vi "Format Spreadsheet Header.vi"(10 "Channel Settings":T1[](array[typedef])) -> (2 "Log file header":string)   [LabVIEW 2021, in "Logging.lvlib"]
doc: "Format a starting timestamp and column headings using the channel names from 'Channel Settings'."
uses:
  Logging.lvlib
  Acquisition/Channel Settings.ctl
  Acquisition/IO Device.ctl
  Acquisition/Acquisition.lvlib
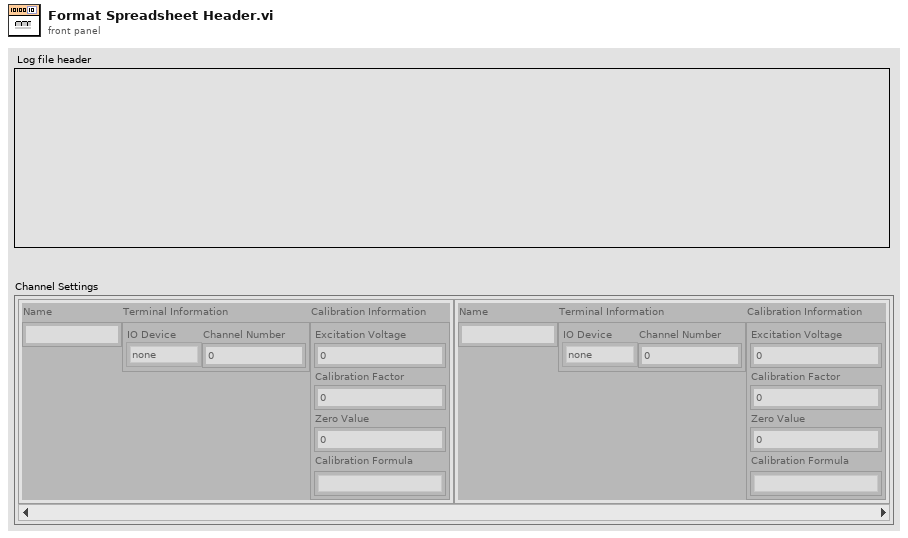
[diagram p1: front panel]
types:
  T1 = typedef "Acquisition.lvlib/Channel Settings.ctl" = cluster{"Name":string, "Terminal Information":cluster{"IO Device":T2, "Channel Number":i32}, "Calibration Information":cluster{"Excitation Voltage":dbl, "Calibration Factor":dbl, "Zero Value":dbl, "Calibration Formula":string}}
  T2 = typedef "Acquisition.lvlib/IO Device.ctl" = enum16{"none", "9219", "9401"}
  T3 = cluster{"Excitation Voltage":dbl, "Calibration Factor":dbl, "Zero Value":dbl, "Calibration Formula":string}
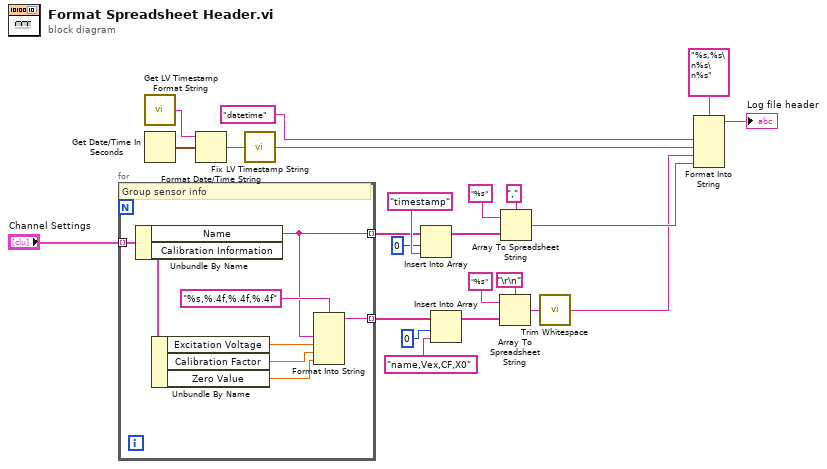
[diagram p0: block diagram]
diagram:
  n1 = for {
    tunnel: "Channel Settings" -> [w31] mode=indexing
    tunnel: [w25] -> w14 mode=indexing
    tunnel: [w24] -> w1 mode=indexing
    # "Group sensor info"
    n2 = Unbundle By Name(w31) -> ("Name"=w24:string, "Calibration Information"=w30:T3)
    n3 = Unbundle By Name(w30) -> ("Excitation Voltage"=w28:dbl, "Calibration Factor"=w27:dbl, "Zero Value"=w26:dbl)
    n4 = Format Into String(format string="%s,%.4f,%.4f,%.4f", w24, w28, w27, w26) -> (resulting string=w25:string)  [unwired: 2 in, 1 out]
  }
  n5 = call "Get LV Timestamp Format String.vi"() -> ("timestamp string format"=w9:string)
  n6 = Get Date/Time In Seconds() -> (seconds since 1Jan1904=w23:timestamp)
  n7 = Format Date/Time String(time format string (%c)=w9, seconds (now)=w23) -> (date/time string=w8:string)  [unwired: 1 in]
  n8 = call "Fix LV Timestamp String.vi"("LabVIEW format string"=w8) -> ("iso 8601 format string"=w5:string)
  n9 = Insert Into Array(array=w1, index=0, new element="timestamp" ("new element/subarray")) -> (w19:string[])
  n10 = Insert Into Array(array=w14, index=0, new element="name,Vex,CF,X0" ("format string")) -> (w11:string[])
  n11 = Array To Spreadsheet String(delimiter (Tab)="\r\n", array=w11, 3:"%s" ("format string")) -> (spreadsheet string=w4:string)
  n12 = Array To Spreadsheet String(delimiter (Tab)=",", array=w19, 3:"%s" ("format string")) -> (spreadsheet string=w3:string)
  n13 = call <vilib>:"Trim Whitespace.vi"("string"=w4) -> ("trimmed string"=w2:string)  [unwired: 1 in]
  n14 = Format Into String(format string="%s,%s\n%s\n%s", "datetime", w5, w2, w3) -> (resulting string=→"Log file header":string)  [unwired: 2 in, 1 out]
